vi "String_parsingV5_time.vi"(5 "input string":string) -> (0 "Time":i32[](array[numeric]), 1 "V2":i32[](array[numeric]), 2 "V3":i32[](array[numeric]), 3 "V1":i32[](array[numeric]))   [LabVIEW 2014]
panel:
  out "size(s)":i32
  out "input test":u8[](array[numeric])
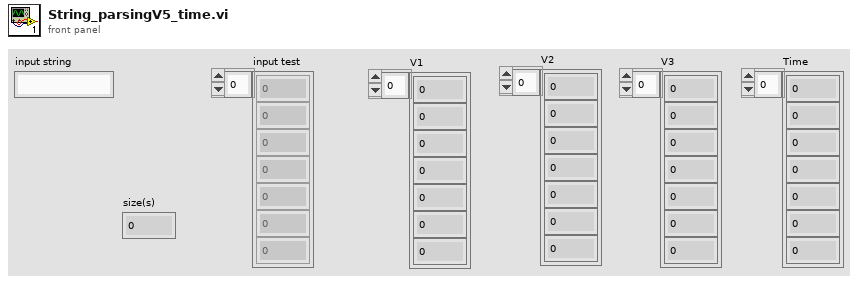
[diagram p1: front panel]
types:
  T1 = typedef "LVDateTimeRec.ctl" = cluster{"fractional second":dbl, "second":i32, "minute":i32, "hour":i32, "day of month":i32, "month":i32, "year":i32, "day of week":i32, "day of year":i32, "DST":i32}
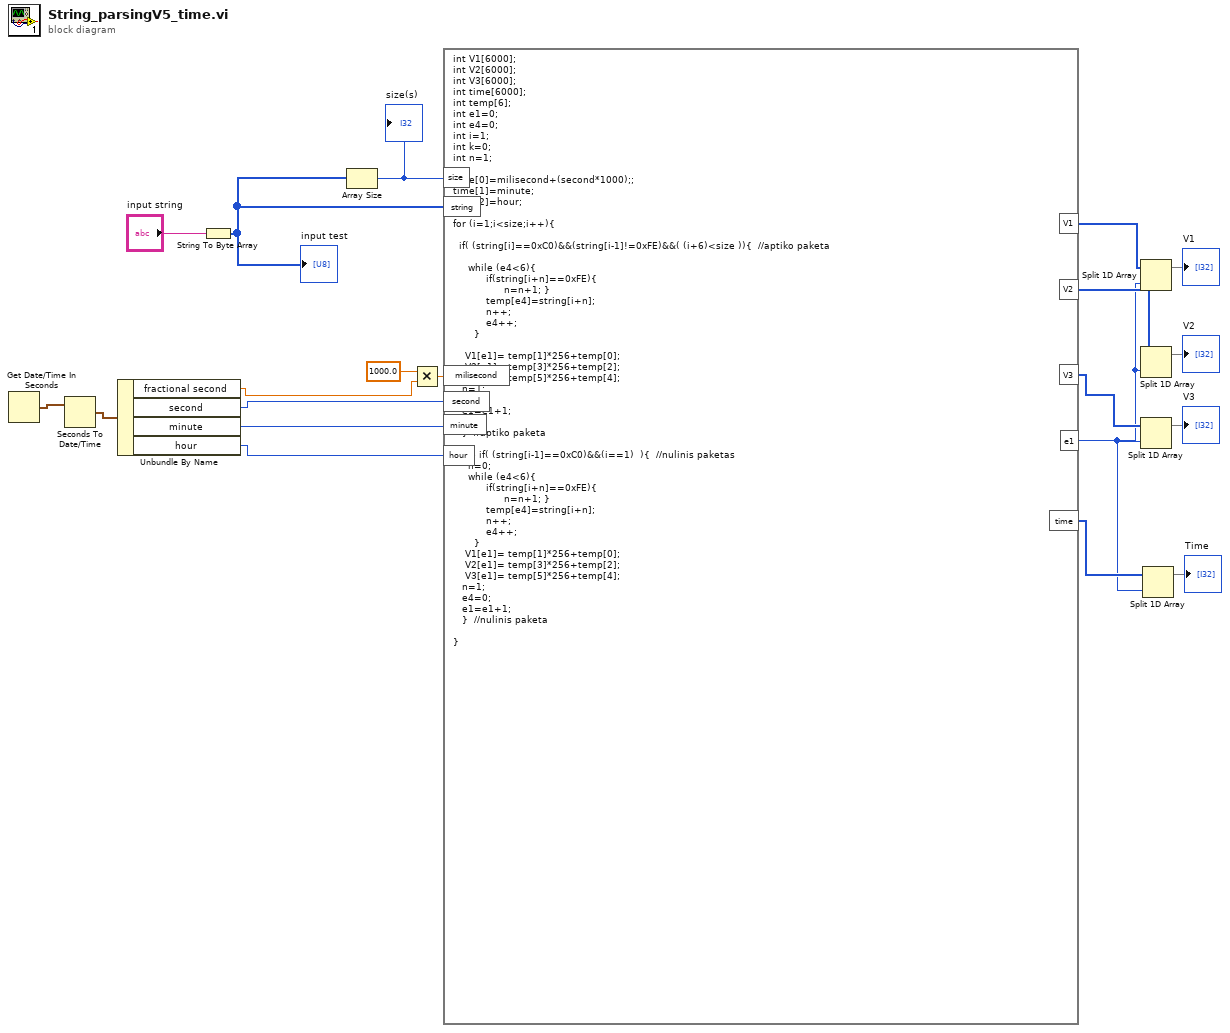
[diagram p0: block diagram]
diagram:
  n1 = Get Date/Time In Seconds() -> (seconds since 1Jan1904=w8:timestamp)
  n2 = Seconds To Date/Time(time stamp (now)=w8) -> (date time rec=w7:T1)  [unwired: 1 in]
  n3 = Unbundle By Name(w7) -> ("fractional second"=w3:dbl, "second"=w6:i32, "minute"=w5:i32, "hour"=w4:i32)
  n4 = String To Byte Array(string="input string") -> (unsigned byte array=w20:u8[])
  "input test" <- w20
  n5 = Array Size(array=w20) -> (size(s)=w19:i32)
  "size(s)" <- w19
  n6 = Multiply(x=1000.0, y=w3) -> (x*y=w1:dbl)
  n7 = formula code="int V1[6000];\nint V2[6000];\nint V3[6000];\nint time[6000];\nint temp[6];\nint e1=0;\nint e4=0;\nint i=1;\nint k=0;\nint n=1;\n\ntime[0]=milisecond+(second*1000);;\ntime[1]=minute;\ntime[2]=hour;\n\nfor (i=1;i<size;i++){\n \n  if( (string[i]==0xC0)&&(string[i-1]!=0xFE)&&( (i+6)<size )){  //aptiko paketa\n\n     while (e4<6){\n           if(string[i+n]==0xFE){\n                 n=n+1; }\n           temp[e4]=string[i+n];\n           n++; \n           e4++;\n       }\n   \n    V1[e1]= temp[1]*256+temp[0];\n    V2[e1]= temp[3]*256+temp[2];\n    V3[e1]= temp[5]*256+temp[4];\n   n=1;\n   e4=0;\n   e1=e1+1;\n   \n   }  //aptiko paketa\n\n else if( (string[i-1]==0xC0)&&(i==1)  ){  //nulinis paketas\n     n=0;\n     while (e4<6){\n           if(string[i+n]==0xFE){\n                 n=n+1; }\n           temp[e4]=string[i+n];\n           n++; \n           e4++;\n       }\n    V1[e1]= temp[1]*256+temp[0];\n    V2[e1]= temp[3]*256+temp[2];\n    V3[e1]= temp[5]*256+temp[4];\n   n=1;\n   e4=0;\n   e1=e1+1;\n   }  //nulinis paketa\n\n}"("string"=w20, "size"=w19, "milisecond"=w1, "second"=w6, "minute"=w5, "hour"=w4) -> ("V1"=w17:i32[], "V2"=w13:i32[], "V3"=w12:i32[], "e1"=w9:i32, "time"=w10:i32[])
  n8 = Split 1D Array(array=w17, index=w9) -> (first subarray=→"V1":i32[])  [unwired: 1 out]
  n9 = Split 1D Array(array=w13, index=w9) -> (first subarray=→"V2":i32[])  [unwired: 1 out]
  n10 = Split 1D Array(array=w12, index=w9) -> (first subarray=→"V3":i32[])  [unwired: 1 out]
  n11 = Split 1D Array(array=w10, index=w9) -> (first subarray=→"Time":i32[])  [unwired: 1 out]
